vi "super small oscilloscope backup.vi"() -> ()   [LabVIEW 2017]
uses:
  <vilib>/Instr/_visa.llb/VISA Set IO Buffer Mask.ctl
  <vilib>/Platform/TimedLoop/XDataNode/timing_clust.ctl
  <vilib>/Platform/TimedLoop/XDataNode/nitl_modes.ctl
  <vilib>/Platform/TimedLoop/XDataNode/wakeup.ctl
  typedefs/commandType.ctl
  <vilib>/Instr/_visa.llb/VISA Configure Serial Port (Instr).vi
  <vilib>/platform/TimedLoop/XDataNode/XDataNode.xnode
  <vilib>/Platform/TimedLoop/XDataNode/XDNodeRunTimeDep.lvlib
panel:
  in  "open files":bool
  in  "close files":bool
  in  "base path":path
  in  "auto fire":bool=TRUE
  in  "pulse duration (ms)":dbl=9.0 format="%#_6f"
  in  "hysteresis (mV)":dbl=50.0 format="%#_6f"
  in  "slope":bool
  in  "pulse phase (deg)":dbl=15.0 format="%#_6p"
  out "gain":dbl
  in  "Gain setting":u8
  in  "LED level":u8(slide) scale=0.0..255.0
  in  "coil on":bool
  out "T":dbl
  in  "pretrigger":dbl
  out "crossing-2":dbl
  in  "trigger":bool
  out "recent crossing":dbl
  out "prev crossing":dbl
  in  "sample length":i32=5000
  out "z accel":dbl format="%0.2f"
  out "Yaccel":dbl(slide) scale=-1.0..1.0
  out "Xaccel":dbl(slide) scale=-1.0..1.0
  in  "reset":bool
  out "deg/hr":dbl format="%0.2f"
  out "angle vs time":cluster{dbl[], dbl[]}[](graph)
  out "angle":dbl
  out "magnet":cluster{dbl[], "Best Linear Fit":dbl[]}[](graph)
  in  "time range (s)":dbl=2.2 format="%#_13g"
  in  "stop 2":bool
  out "voltage":cluster{dbl[], dbl[]}[](graph)
  out "error out":errorcluster
  in  "stop":bool
  in  "VISA resource name":refnum<visa-resource-name>
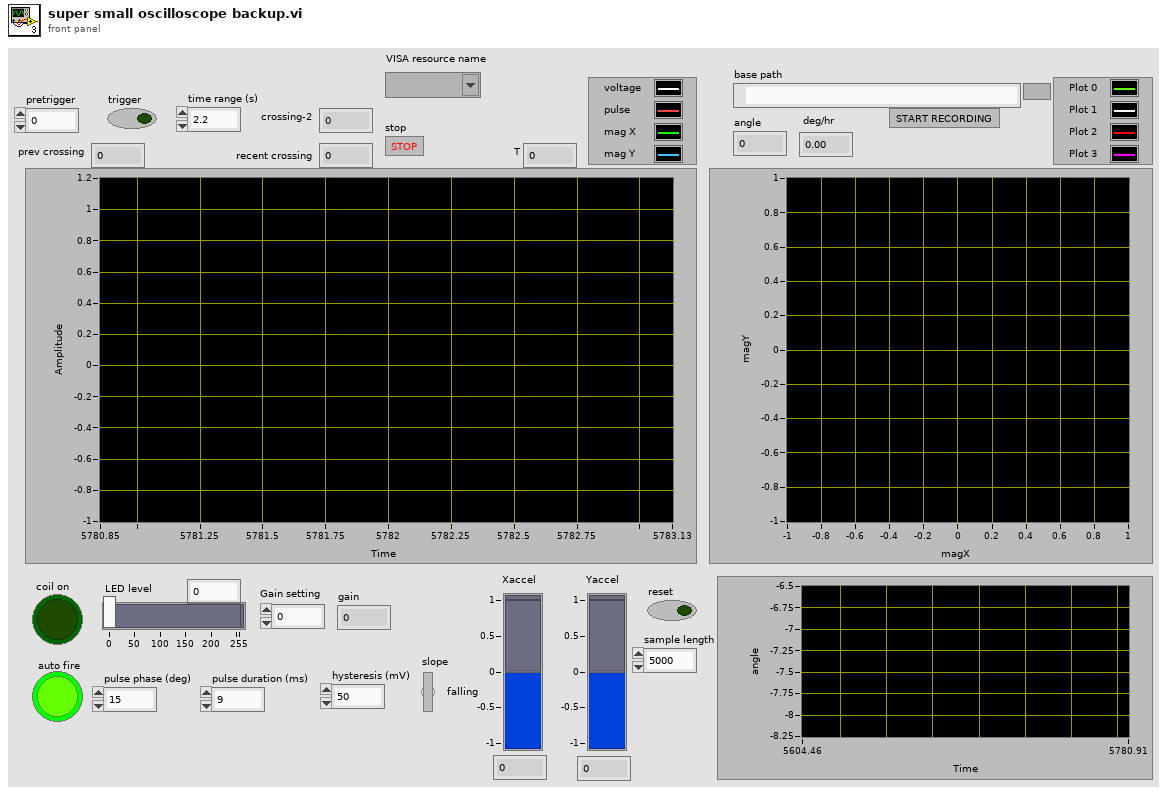
[diagram p1: front panel]
types:
  T1 = typedef "VISA Set IO Buffer Mask.ctl" = u16
  T2 = cluster{"voltage":refnum<queue>, "coil":refnum<queue>, "mag":refnum<queue>, "accel":refnum<queue>}
  T3 = typedef "commandType.ctl" = enum16{"G - set gain", "C - activate coil", "D - deactivate coil", "L - set LED", "A - set AUTO", "V - set verbose"}
  T4 = typedef "XDNodeRunTimeDep.lvlib/timing_clust.ctl" = cluster{"Expected End [f-1]":u64, "Actual End [f-1]":u64, "Finished Late? [f-1]":bool, "Expected End [i-1]":u64, "Actual End [i-1]":u64, "Finished Late? [i-1]":bool, "Expected Start [i]":u64, "Actual Start [i]":u64, "Expected Start [f]":u64, "Actual Start [f]":u64, "Source Name":string, "Structure Name":string, "Period":i64, "Deadline":i64, "Offset":i64, "Start":i64, "Priority":i32, "Timeout":i32, "Mode":T5, "Wakeup Reason":T6, "Error":errorcluster, "Source Type":string, "Secondary Source Type":string, "Global End Time":u64, "Global Start Time":u64, "Frame Duration":u64, "Iteration Duration":u64, "Assigned CPU":i32, "I/O Scan Engine Mode":u32}
  T5 = typedef "XDNodeRunTimeDep.lvlib/nitl_modes.ctl" = enum32{"No Change", "Process missed periods, maintain original phase", "Discard missed periods, maintain original phase", "Process missed periods, ignore original phase", "Discard missed periods, ignore original phase"}
  T6 = typedef "XDNodeRunTimeDep.lvlib/wakeup.ctl" = enum32{"Normal", "Aborted", "Asynchronous wakeup", "Timing source error", "Timed loop error", "Timeout"}
  T7 = cluster{"voltage file":refnum<file>, "coil file":refnum<file>, "mag file":refnum<file>}
  T8 = cluster{"Best Linear Fit":dbl[], "Best Linear Fit":dbl[]}[]
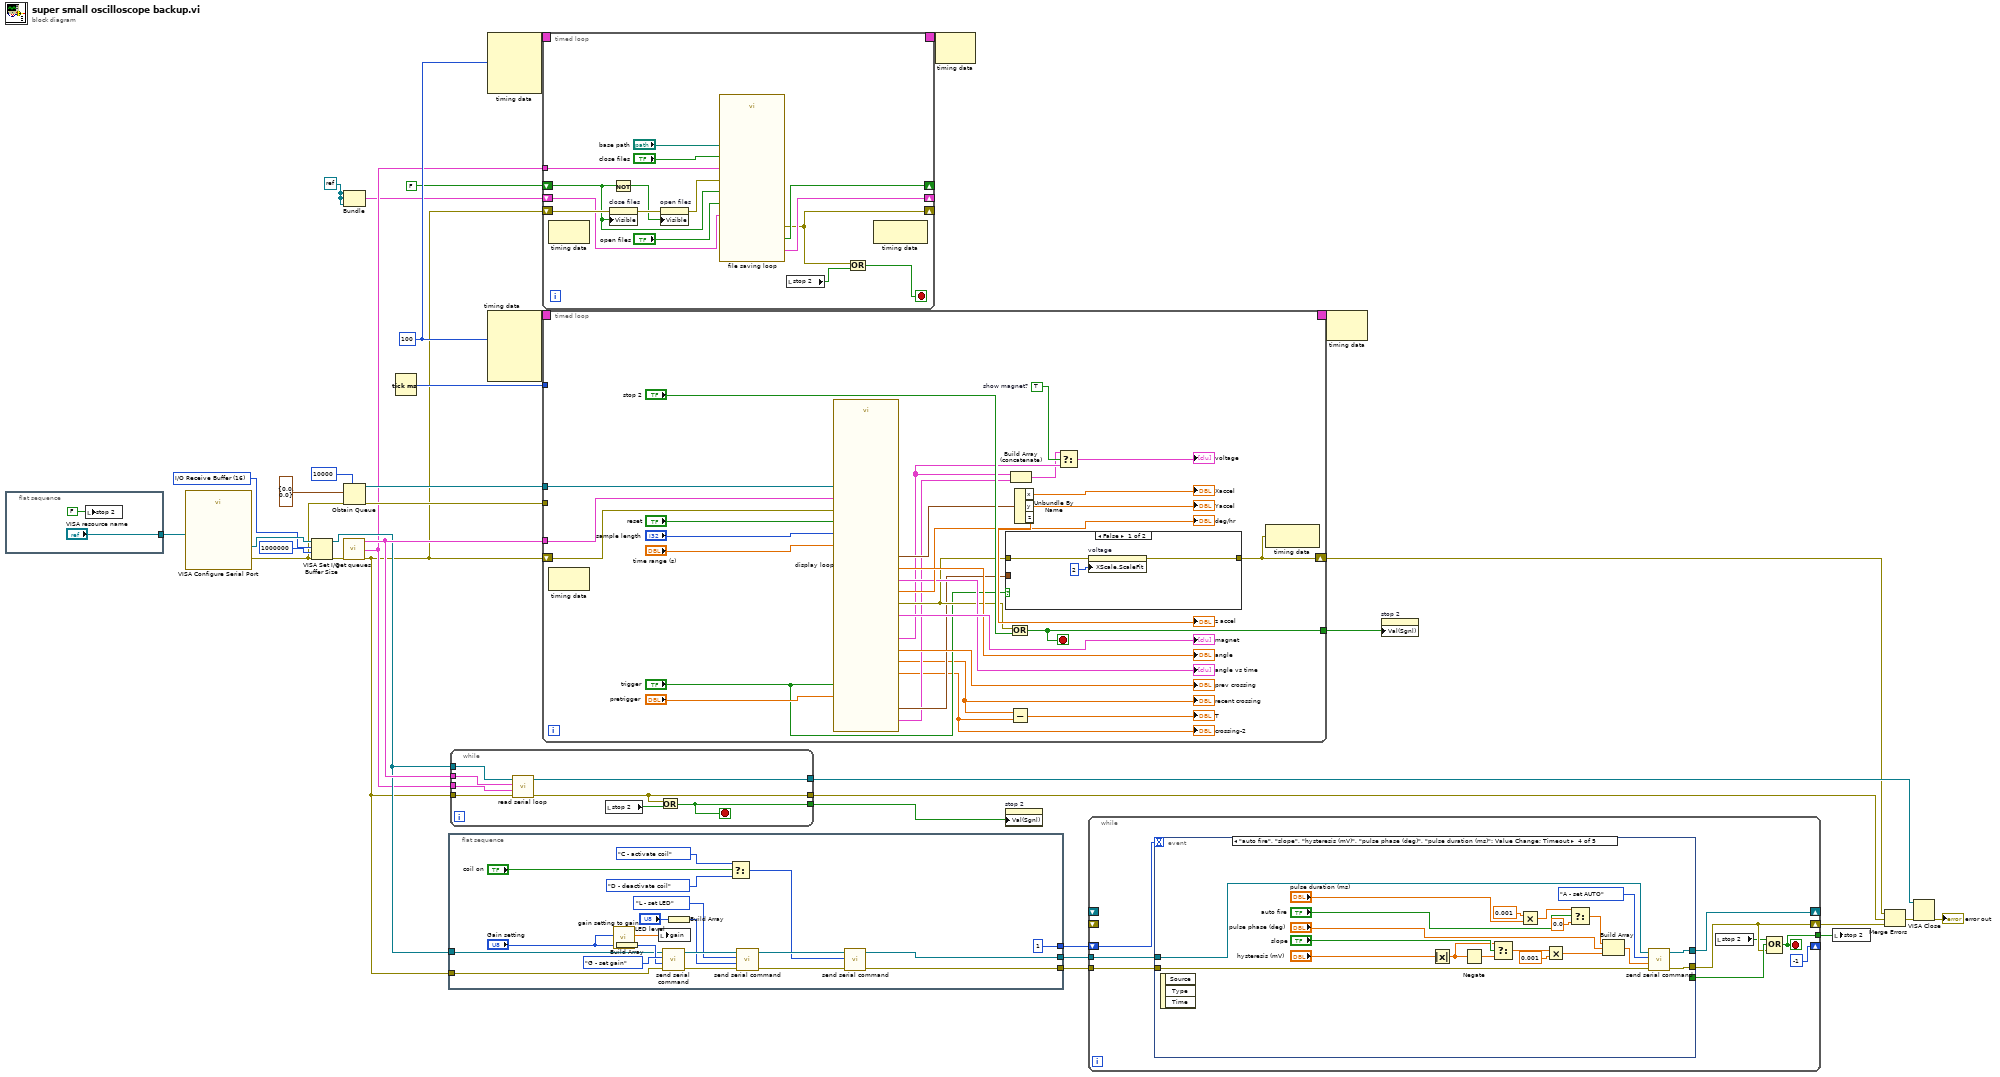
[diagram p0: block diagram]
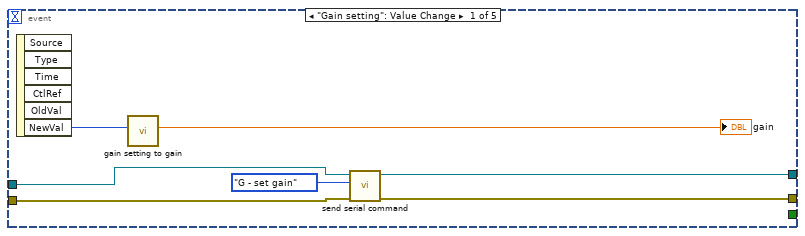
[diagram p2: hidden frame]
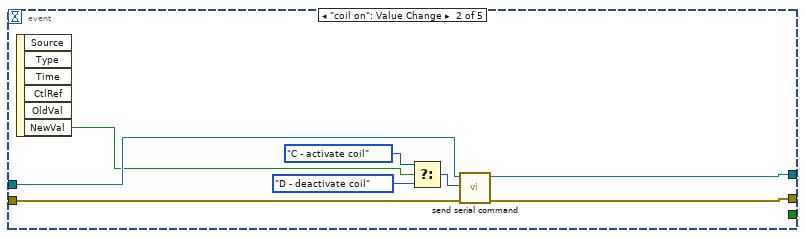
[diagram p3: hidden frame]
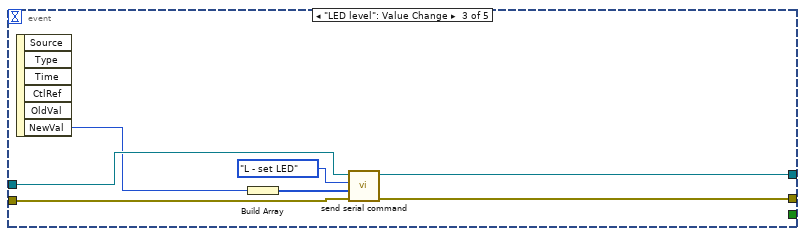
[diagram p4: hidden frame]
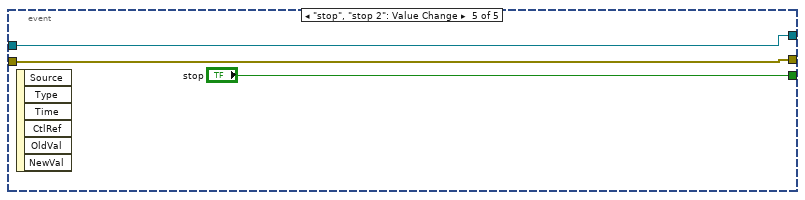
[diagram p5: hidden frame]
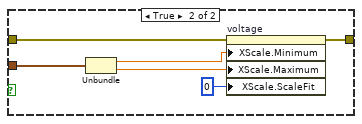
[diagram p6: hidden frame]
diagram:
  w2 = refnum<k0> refnum
  w6 = i64 100 ("update (ms)")
  w33 = T1 16 items=["I/O Receive Buffer"=16, "I/O Transmit Buffer"=32, "I/O Receive and Transmit Buffer"=48] ("Mask")
  n1 = flat-sequence {
    tunnel: ["VISA resource name"] -> w20
    frame #0 {
      n2 = local write "stop 2"(FALSE ("stop 2")) -> ()
    }
  }
  n3 = call-poly "VISA Configure Serial Port"("VISA resource name"=w20) -> ("VISA resource name out"=w35:refnum<visa-resource-name>, "error out"=w19:errorcluster)  [unwired: 13 in]
  n4 = VISA Set I/O Buffer Size(VISA resource name=w35, mask (16)=w33, size (4096)=u32 1000000, error in (no error)=w19) -> (VISA resource name out=w14:refnum<visa-resource-name>, error out=w22:errorcluster)
  n5 = call "get queues.vi"("error in (no error)"=w22) -> ("display queues"=w21:T2, "disk queues"=w5:T2, "error out"=w4:errorcluster)  [unwired: 12 in]
  n6 = Bundle(w2, w2, w2) -> (w1:cluster{refnum<k0>, refnum<k0>, refnum<k0>})  [unwired: 1 in]
  n7 = Obtain Queue(max queue size (-1, unlimited)=10000, element data type=cluster{"mean":dbl, dbl} {"mean"=0.0, 0.0} ("output cluster"), error in (no error)=w19) -> (queue out=w25:refnum<queue>, error out=w24:errorcluster)  [unwired: 2 in, 1 out]
  n8 = Tick Count (ms)() -> (millisecond timer value=w27:u32)
  n9 = flat-sequence {
    tunnel: [w53] -> w18
    tunnel: [w52] -> w17
    tunnel: [1] -> w16
    tunnel: w4 -> [w39]
    tunnel: w14 -> [w38]
    frame #0 {
      n10 = call "gain setting to gain.vi"("Gain setting"="Gain setting") -> ("gain"=w48:dbl)  [unwired: 10 in]
      n11 = Build Array("Gain setting") -> (w50:u8[])
      n12 = local write "gain"(w48) -> ()
      n13 = call "send serial command.vi"("error in (no error)"=w39, "data"=w50, "Command"=commandType."G - set gain", "visa resource"=w38) -> ("error out"=w57:errorcluster, "VISA resource name out"=w56:refnum<visa-resource-name>)  [unwired: 6 in]
      n14 = Build Array("LED level") -> (w46:u8[])
      n15 = Select(t=commandType."C - activate coil" ("Command"), s="coil on", f=commandType."D - deactivate coil") -> (s? t:f=w41:T3)
      n16 = call "send serial command.vi"("error in (no error)"=w57, "data"=w46, "Command"=commandType."L - set LED", "visa resource"=w56) -> ("error out"=w54:errorcluster, "VISA resource name out"=w55:refnum<visa-resource-name>)  [unwired: 6 in]
      n17 = call "send serial command.vi"("error in (no error)"=w54, "Command"=w41, "visa resource"=w55) -> ("error out"=w52:errorcluster, "VISA resource name out"=w53:refnum<visa-resource-name>)  [unwired: 7 in]
    }
  }
  n18 = while {
    tunnel: w4 -> [w65]
    tunnel: w21 -> [w64]
    tunnel: w5 -> [w63]
    tunnel: w14 -> [w62]
    tunnel: [w61] -> w30
    tunnel: [w60] -> w29
    tunnel: [w59] -> w12
    stop <- w59 stop-if-true
    n19 = call "read serial loop.vi"("error in (no error)"=w65, "disk queues"=w63, "display queues"=w64, "serial port"=w62) -> ("error out"=w60:errorcluster, "VISA resource name out"=w61:refnum<visa-resource-name>)  [unwired: 6 in]
    n20 = local read "stop 2"() -> (w58:bool)
    n21 = Or(x=w60, y=w58) -> (x .or. y?=w59:bool)
  }
  n22 = node-c288(w6) -> (w8:T4)  [unwired: 3 in]
  n23 = node-c288(w6) -> (w32:T4)  [unwired: 4 in]
  n24 = timed-loop {
    timing: w8 -> [_]
    timing-out: [_] -> w7
    tunnel: w5 -> [w77]
    shift-right: [w76] -> _
    shift-left: FALSE ("files open out") -> [w72]
    shift-right: [w68] -> _
    shift-left: w4 -> [w75]
    shift-right: [w70] -> _
    shift-left: w1 -> [w69]
    stop <- w66 stop-if-true
    n25 = node-c288() -> ()  [unwired: 1 in, 1 out]
    n26 = property on="close files" class="Bool (strict)"(error in=w75, "Visible"=w72) -> (error out=w74:errorcluster)  [unwired: 1 in, 1 out]
    n27 = Not(x=w72) -> (.not. x?=w71:bool)
    n28 = property on="open files" class="Bool"(error in=w74, "Visible"=w71) -> (error out=w73:errorcluster)  [unwired: 1 in, 1 out]
    n29 = call "file saving loop.vi"("files open"=w72, "refnums"=w69, "disk queues"=w77, "close files"="close files", "open files"="open files", "error in"=w73, "base path"="base path") -> ("files open out"=w76:bool, "refnums out"=w70:T7, "error out"=w68:errorcluster)  [unwired: 10 in]
    n30 = local read "stop 2"() -> (w67:bool)
    n31 = Or(x=w68, y=w67) -> (x .or. y?=w66:bool)
    n32 = node-c288() -> ()  [unwired: 1 in, 1 out]
  }
  n33 = timed-loop {
    timing: w32 -> [_]
    timing-out: [_] -> w31
    tunnel: w27 -> [_]
    shift-right: [w92] -> w9
    shift-left: w4 -> [w107]
    tunnel: w25 -> [w106]
    tunnel: w24 -> [_]
    tunnel: w21 -> [w111]
    tunnel: [w83] -> w13
    stop <- w83 stop-if-true
    w91 = TRUE  # show magnet?
    n34 = node-c288() -> ()  [unwired: 1 in, 1 out]
    n35 = call "display loop.vi"("display queues"=w111, "sample length"="sample length", "reset"="reset", "time range (s)"="time range (s)", "angle queue"=w106, "error in"=w107, "trigger"="trigger", "pretrigger"="pretrigger") -> ("crossing-2"=w85:dbl, "magnet vs time"=w89:cluster{dbl[], dbl[]}[], "recent crossing"=w86:dbl, "trigger x-axis"=w94:cluster{dbl, dbl}, "prev crossing"=→"prev crossing":dbl, "angle"=→"angle":dbl, "deg/hr"=→"deg/hr":dbl, "accel"=w105:cluster{"x":dbl, "y":dbl, "z":dbl}, "angle graph"=→"angle vs time":cluster{dbl[], dbl[]}[], "voltage graphs"=w88:cluster{dbl[], dbl[]}[], "magnet graphs"=→"magnet":T8, "error out"=w97:errorcluster)  [unwired: 7 in, 1 out]
    "recent crossing" <- w86
    "crossing-2" <- w85
    n36 = case shown="False" "trigger" {
      tunnel: w97 -> [w115 w121]
      tunnel: w94 -> [_ w120]
      tunnel: [w113 w117] -> w92
      frame False {
        n37 = property on="voltage" class="XYGraph (strict)"(error in=w115, "XScale.ScaleFit"=u8 2 ("X Scale.Scale Fit")) -> (error out=w113:errorcluster)  [unwired: 1 in, 1 out]
      }
      frame True {
        n38 = Unbundle(w120) -> (w119:dbl, w118:dbl)
        n39 = property on="voltage" class="XYGraph (strict)"(error in=w121, "XScale.Minimum"=w119, "XScale.Maximum"=w118, "XScale.ScaleFit"=u8 0 ("X Scale.Scale Fit")) -> (error out=w117:errorcluster)  [unwired: 1 in, 1 out]
      }
    }
    n40 = Or(x=w97, y="stop 2") -> (x .or. y?=w83:bool)
    n41 = Subtract(x=w86, y=w85) -> (x-y=→"T":dbl)
    n42 = Build Array (concatenate)(w88, w89) -> (w87:cluster{dbl[], dbl[]}[])
    n43 = Unbundle By Name(w105) -> ("x"=→"Xaccel":dbl, "y"=→"Yaccel":dbl, "z"=→"z accel":dbl)
    n44 = Select(t=w87, s=w91, f=w88) -> (s? t:f=→"voltage":cluster{dbl[], dbl[]}[])
    n45 = node-c288(w92) -> ()  [unwired: 1 out]
  }
  n46 = node-c288(w7) -> ()  [unwired: 1 out]
  n47 = property on="stop 2" class="Bool (strict)"("Val(Sgnl)"=w12) -> ()  [unwired: 2 in, 2 out]
  n48 = while {
    tunnel: w18 -> [w134]
    tunnel: w17 -> [w133]
    shift-right: [w131] -> _
    shift-left: _ -> [_]
    shift-right: [w128] -> w10
    shift-left: _ -> [_]
    shift-right: [-1] -> _
    shift-left: w16 -> [w132]
    tunnel: [w127] -> w15
    stop <- w127 stop-if-true
    n49 = event shown="[3] \"auto fire\", \"slope\", \"hysteresis (mV)\", \"pulse phase (deg)\", \"pulse duration (ms)\": Value Change;  Timeout" {
      selector: _ -> [_ _ _ _ _]
      dyn-events: _ -> [_ _ _ _ _]
      timeout: w132 -> [_ _ _ _ _]
      tunnel: w134 -> [w140 w149 w156 w176 w178]
      tunnel: w133 -> [w138 w148 w154 w174 w179]
      tunnel: [w137 w147 w153 w173 w178] -> w131
      tunnel: [w136 w146 w152 w172 w179] -> w128
      tunnel: [_ _ _ _ "stop"] -> w129
      event "Gain setting": Value Change {
        n50 = event-data() -> ("NewVal"=w135:u8)  [unwired: 1 in, 5 out]
        n51 = call "gain setting to gain.vi"("Gain setting"=w135) -> ("gain"=→"gain":dbl)  [unwired: 10 in]
        n52 = call "send serial command.vi"("error in (no error)"=w138, "Command"=commandType."G - set gain", "visa resource"=w140) -> ("error out"=w136:errorcluster, "VISA resource name out"=w137:refnum<visa-resource-name>)  [unwired: 7 in]
      }
      event "coil on": Value Change {
        n53 = event-data() -> ("NewVal"=w143:bool)  [unwired: 1 in, 5 out]
        n54 = Select(t=commandType."C - activate coil" ("Command"), s=w143, f=commandType."D - deactivate coil") -> (s? t:f=w142:T3)
        n55 = call "send serial command.vi"("error in (no error)"=w148, "Command"=w142, "visa resource"=w149) -> ("error out"=w146:errorcluster, "VISA resource name out"=w147:refnum<visa-resource-name>)  [unwired: 7 in]
      }
      event "LED level": Value Change {
        n56 = event-data() -> ("NewVal"=w151:u8)  [unwired: 1 in, 5 out]
        n57 = Build Array(w151) -> (w150:u8[])
        n58 = call "send serial command.vi"("error in (no error)"=w154, "data"=w150, "Command"=commandType."L - set LED", "visa resource"=w156) -> ("error out"=w152:errorcluster, "VISA resource name out"=w153:refnum<visa-resource-name>)  [unwired: 6 in]
      }
      event "auto fire", "slope", "hysteresis (mV)", "pulse phase (deg)", "pulse duration (ms)": Value Change; Timeout {
        n59 = event-data() -> ()  [unwired: 1 in, 3 out]
        n60 = Absolute Value(x="hysteresis (mV)") -> (abs(x)=w166:dbl)
        n61 = Negate(x=w166) -> (-x=w165:dbl)
        n62 = Select(t=w166, s="slope", f=w165) -> (s? t:f=w162:dbl)
        n63 = Multiply(x=0.001, y="pulse duration (ms)") -> (x*y=w158:dbl)
        n64 = Multiply(x=w162, y=0.001) -> (x*y=w160:dbl)
        n65 = Select(t=w158, s="auto fire", f=0.0) -> (s? t:f=w164:dbl)
        n66 = Build Array(w164, "pulse phase (deg)", w160) -> (w161:dbl[])
        n67 = call "send serial command.vi"("error in (no error)"=w174, "data"=w161, "Command"=commandType."A - set AUTO", "visa resource"=w176) -> ("error out"=w172:errorcluster, "VISA resource name out"=w173:refnum<visa-resource-name>)  [unwired: 6 in]
      }
      event "stop", "stop 2": Value Change {
        n68 = event-data() -> ()  [unwired: 1 in, 6 out]
      }
    }
    n69 = local read "stop 2"() -> (w126:bool)
    n70 = Compound Arithmetic op=OR(w126, w129, w128) -> (w127:bool)
  }
  n71 = node-c288(w31) -> ()  [unwired: 1 out]
  n72 = property on="stop 2" class="Bool (strict)"("Val(Sgnl)"=w13) -> ()  [unwired: 2 in, 2 out]
  n73 = local write "stop 2"(w15) -> ()
  n74 = Merge Errors(w9, w29, w10) -> (w11:errorcluster)
  n75 = VISA Close(VISA resource name=w30, error in (no error)=w11) -> (error out=→"error out":errorcluster)
